vi "SaveTwoHands.vi"(8 "error in (no error)":errorcluster, 11 "Controller Refnum":refnum<k24>) -> (0 "error out":errorcluster, 3 "Hand array":T1[](array[typedef]))   [LabVIEW 2017, in "LeapMotion.lvlib"]
uses:
  LeapMotion.lvlib
  TypeDefs/LEAPhand.ctl
  TypeDefs/LEAParm.ctl
  TypeDefs/LEAPvector.ctl
  TypeDefs/LEAPfinger.ctl
  TypeDefs/LEAPbone.ctl
  C:/Users/Sara/Documents/GitHub/LEAP-sign-language/LEAP-sign-language/LeapMotion/Dynamic Libraries/LeapCSharp.NET4.5.dll
  Dynamic Libraries/LeapCSharp.NET4.5.dll
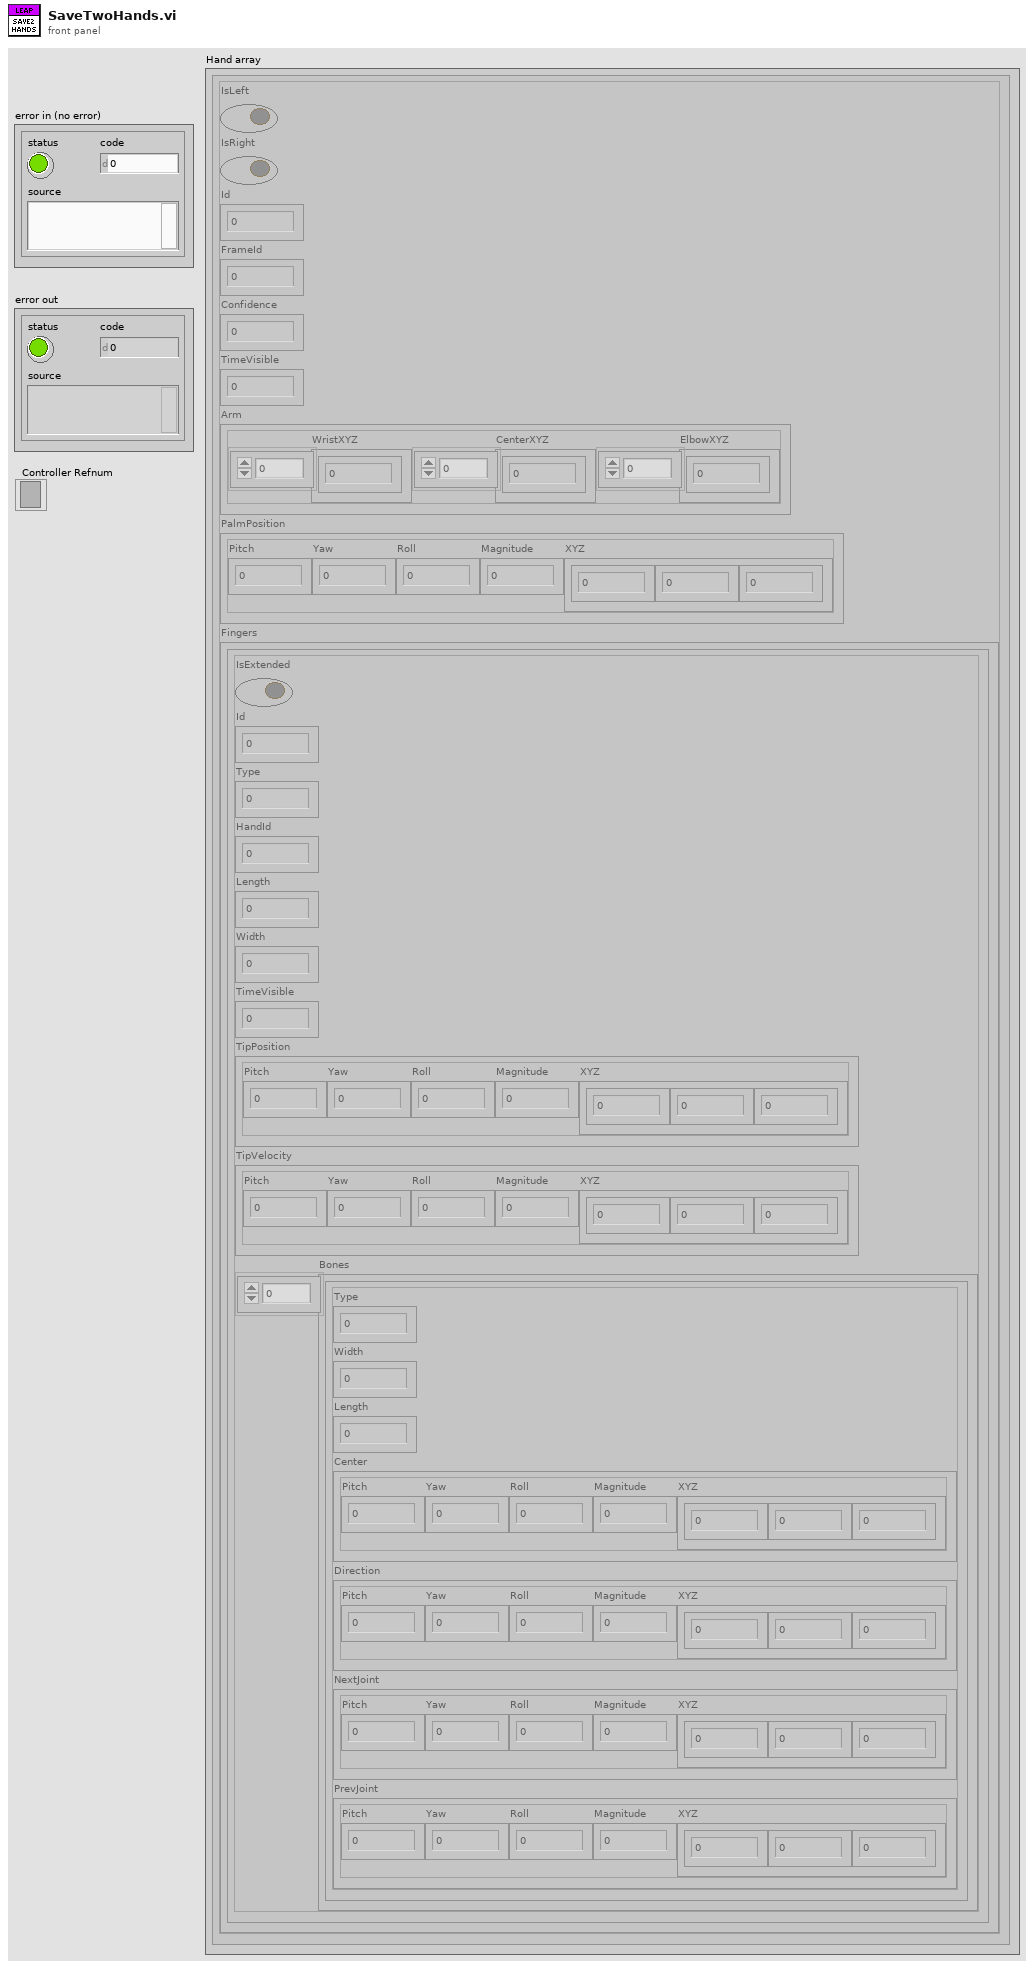
[diagram p1: front panel]
types:
  T1 = typedef "LeapMotion.lvlib/LEAPhand.ctl" = cluster{"IsLeft":bool, "IsRight":bool, "Id":i32, "FrameId":i64, "Confidence":sgl, "TimeVisible":sgl, "Arm":T2, "PalmPosition":T3, "Fingers":T4[]}
  T2 = typedef "LeapMotion.lvlib/LEAParm.ctl" = cluster{"WristXYZ":sgl[], "CenterXYZ":sgl[], "ElbowXYZ":sgl[]}
  T3 = typedef "LeapMotion.lvlib/LEAPvector.ctl" = cluster{"Pitch":sgl, "Yaw":sgl, "Roll":sgl, "Magnitude":sgl, "XYZ":sgl[]}
  T4 = typedef "LeapMotion.lvlib/LEAPfinger.ctl" = cluster{"IsExtended":bool, "Id":i32, "Type":i32, "HandId":i32, "Length":sgl, "Width":sgl, "TimeVisible":sgl, "TipPosition":T3, "TipVelocity":T3, "Bones":T5[]}
  T5 = typedef "LeapMotion.lvlib/LEAPbone.ctl" = cluster{"Type":i32, "Width":sgl, "Length":sgl, "Center":T3, "Direction":T3, "NextJoint":T3, "PrevJoint":T3}
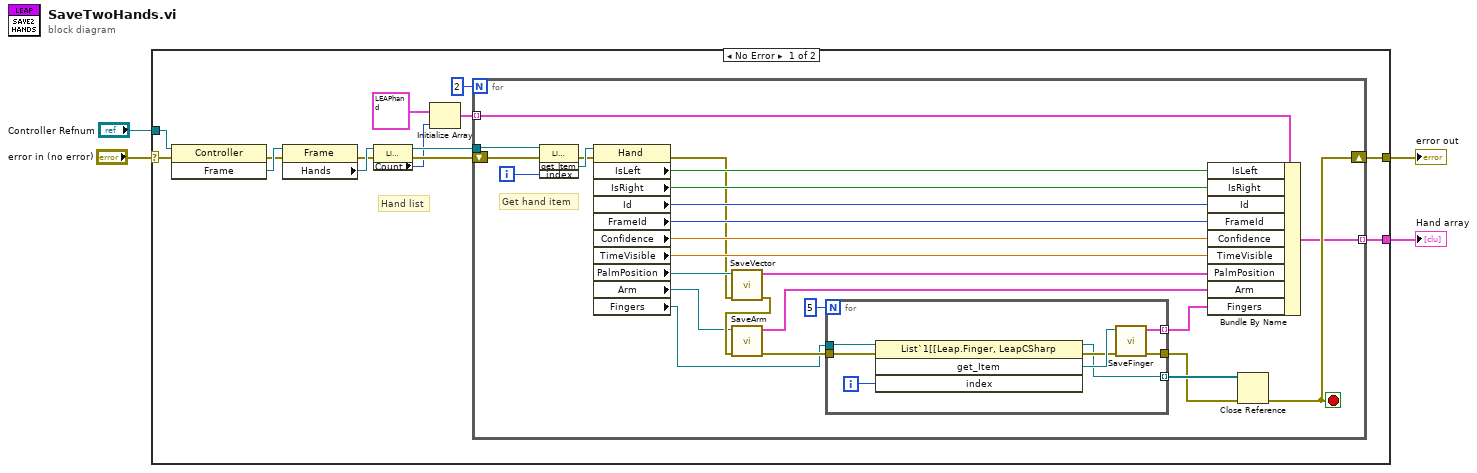
[diagram p0: block diagram]
diagram:
  n1 = case shown="No Error" "error in (no error)" {
    selector: "error in (no error)" -> [w9 w53]
    tunnel: [w16 w53] -> w2
    tunnel: [w13 _] -> w4
    tunnel: "Controller Refnum" -> [w11 _]
    frame No Error {
      # "Hand list"
      n2 = invoke class="Controller" method="Frame"(reference=w11, error in=w9) -> (error out=w8:errorcluster, "Frame"=w12:refnum<k24>)  [unwired: 1 in, 1 out]
      n3 = property class="Frame"(reference=w12, error in=w8) -> (error out=w7:errorcluster, "Hands"=w10:refnum<k24>)  [unwired: 1 out]
      n4 = property class="List`1[[Leap.Hand, LeapCSharp.N"(reference=w10, error in=w7) -> (reference out=w18:refnum<k24>, error out=w17:errorcluster, "Count"=w6:i32)
      n5 = Initialize Array(T1 {"IsLeft"=FALSE, "IsRight"=FALSE, "Id"=0, "FrameId"=0, "Confidence"=0.0, "TimeVisible"=0.0, "Arm"={"WristXYZ"=[], "CenterXYZ"=[], "ElbowXYZ"=[]}, "PalmPosition"={"Pitch"=0.0, "Yaw"=0.0, "Roll"=0.0, "Magnitude"=0.0, "XYZ"=[]}, "Fingers"=[]} ("Hand"), w6) -> (w14:T1[])
      n6 = for {
        N: 2 -> [_]
        tunnel: w18 -> [w44]
        tunnel: w14 -> [w32] mode=indexing
        tunnel: [w27] -> w13 mode=indexing
        shift-right: [w29] -> w16
        shift-left: w17 -> [w43]
        i -> [w28]
        stop <- w29 stop-if-true
        # "Get hand item"
        n7 = invoke class="List`1[[Leap.Hand, LeapCSharp.N" method="get_Item"(reference=w44, error in=w43, "index"=w28) -> (error out=w41:errorcluster, "get_Item"=w42:refnum<k24>)  [unwired: 1 in, 2 out]
        n8 = property class="Hand"(reference=w42, error in=w41) -> (error out=w25:errorcluster, "IsLeft"=w40:bool, "IsRight"=w39:bool, "Id"=w38:i32, "FrameId"=w37:i64, "Confidence"=w36:sgl, "TimeVisible"=w35:sgl, "PalmPosition"=w26:refnum<k24>, "Arm"=w22:refnum<k24>, "Fingers"=w21:refnum<k24>)  [unwired: 1 out]
        n9 = call "SaveVector.vi"("error in (no error)"=w25, "Vector Refnum"=w26) -> ("error out"=w24:errorcluster, "LEAPvector"=w34:T3)  [unwired: 8 in]
        n10 = call "SaveArm.vi"("Error In"=w24, ".NET Refnum in"=w22) -> ("Error Out"=w23:errorcluster, "LEAParm"=w19:T2)  [unwired: 8 in]
        n11 = for {
          N: 5 -> [_]
          tunnel: [w52] -> w30
          tunnel: w21 -> [w49]
          tunnel: [w48] -> w20 mode=indexing
          tunnel: w23 -> [w46]
          tunnel: [w45] -> w31 mode=indexing
          i -> [w47]
          n12 = invoke class="List`1[[Leap.Finger, LeapCSharp" method="get_Item"(reference=w49, error in=w46, "index"=w47) -> (reference out=w45:refnum<k24>, error out=w50:errorcluster, "get_Item"=w51:refnum<k24>)  [unwired: 1 in, 1 out]
          n13 = call "SaveFinger.vi"("error in (no error)"=w50, "Finger Refnum"=w51) -> ("error out"=w52:errorcluster, "Finger"=w48:T4)  [unwired: 8 in]
        }
        n14 = Bundle By Name(cluster=w32, "IsLeft"=w40, "IsRight"=w39, "Id"=w38, "FrameId"=w37, "Confidence"=w36, "TimeVisible"=w35, "PalmPosition"=w34, "Arm"=w19, "Fingers"=w20) -> (w27:T1)
        n15 = Close Reference(reference=w31, error in (no error)=w30) -> (error out=w29:errorcluster)
      }
    }
    frame Error {
    }
  }
  "Hand array" <- w4
  "error out" <- w2
